vi "Config.vi"(8 "error in (no error)":errorcluster, 10 "Setting":variant, 11 "KE27XX DMM in":refnum<class "Keithley 27XX DMM.lvclass">) -> (0 "error out":errorcluster, 3 "KE27XX DMM out":refnum<class "Keithley 27XX DMM.lvclass">)   [LabVIEW 2025, in "DMM.lvlib" / "Keithley 27XX DMM.lvclass"]
uses:
  Keithley 27XX DMM.lvclass
  C:/Users/Public/Documents/Sandia National Labs/TSS Plugin/CEF.lvlibp/Node/CEF_Node.lvclass
  C:/Working copy/tss/Plugin/Engines/DMM/DMM Instrument/DMM Instrument.lvclass
  C:/Users/Public/Documents/Sandia National Labs/TSS Plugin/Abstract Engine.lvlibp/Abstract Instrument/Abstract Instrument.lvclass
  DMM configuration/DMM configuration.lvclass
  Keithley 27XX DMM.lvclass/Keithley 27XX DMM.ctl
  DMM configuration/DMM configuration.lvclass/DMM configuration.ctl
  DMM Channel/DMM Channel.lvclass
  Users/Public/Documents/Sandia National Labs/TSS Plugin/Abstract Engine.lvlibp/Abstract Instrument/Channel.ctl
  Users/Public/Documents/Sandia National Labs/TSS Plugin/Abstract Engine.lvlibp/Channel configuration/Channel configuration.lvclass
  DMM configuration/Read DMM Setting.vi
  Users/Public/Documents/Sandia National Labs/TSS Plugin/CEF.lvlibp/Node/ReadChildren.vi
  Users/Public/Documents/Sandia National Labs/TSS Plugin/Abstract Engine.lvlibp/Channel configuration/Read Channel Setting.vi
  Users/Public/Documents/Sandia National Labs/TSS Plugin/CEF.lvlibp/Node/CEF_Node.lvclass
  Users/Public/Documents/Sandia National Labs/TSS Plugin/CEF.lvlibp/serializable configuration/CEF_serializable configuration.lvclass
  <instrlib>/Keithley 27XX/Keithley 27XX.lvlib
  Users/Public/Documents/Sandia National Labs/TSS Plugin/Abstract Engine.lvlibp/Abstract Instrument/Abstract Instrument.lvclass
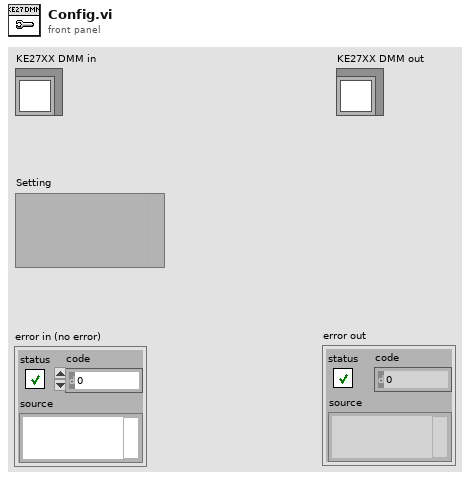
[diagram p1: front panel]
types:
  T1 = typedef "DMM.lvlib/DMM configuration.lvclass/DMM Setting.ctl" = cluster{"Function":string, "CurrentSource":string, "Resolution":string, "Range":dbl}
  T2 = typedef "Abstract Engine.lvlibp/Abstract Instrument.lvclass/Channel.ctl" = cluster{"Alias":string, "DataType":enum16{"Anaolg Input", "Waveform"}, "Unit":enum16{"---", "V", "A", "Ohm", "Hz", "uF", "degC", "deg"}, "Upper limit":dbl, "Lower limit":dbl, "Measurement":variant}
  T3 = typedef "Abstract Engine.lvlibp/Channel configuration.lvclass/Default Channel.ctl" = cluster{"Address":string, "SW Alias":string, "Enabled":bool, "Type":string, "Description":string}
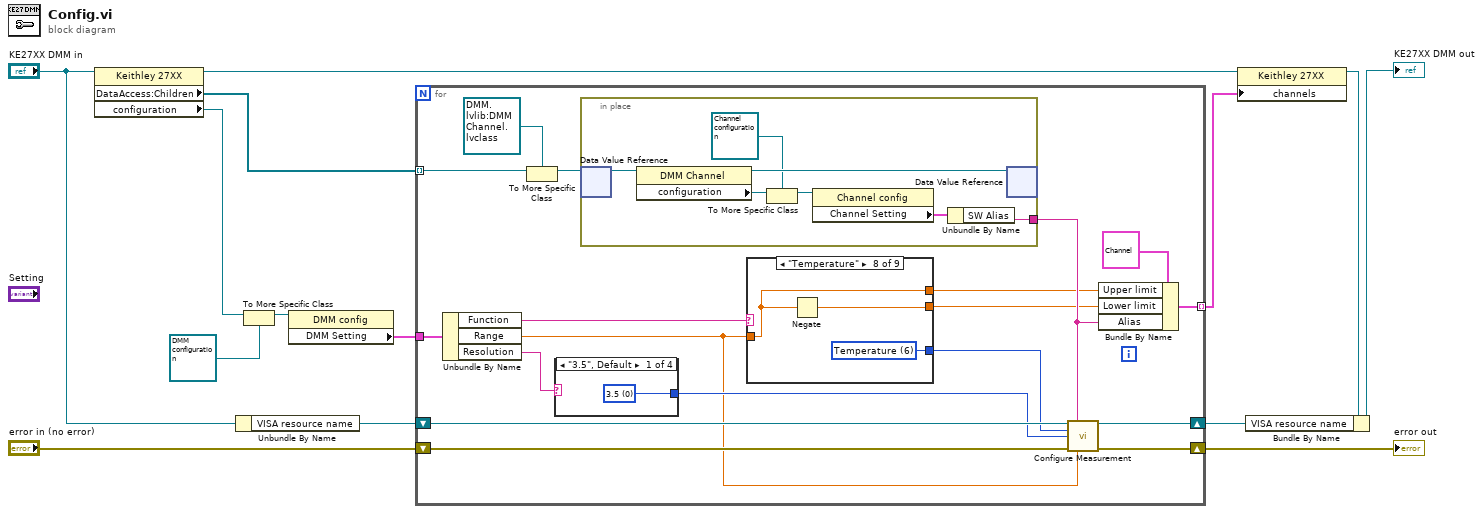
[diagram p0: block diagram]
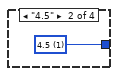
[diagram p2: hidden frame]
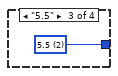
[diagram p3: hidden frame]
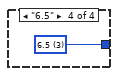
[diagram p4: hidden frame]
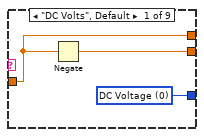
[diagram p5: hidden frame]
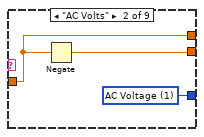
[diagram p6: hidden frame]
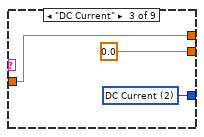
[diagram p7: hidden frame]
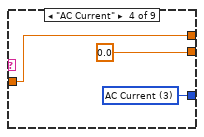
[diagram p8: hidden frame]
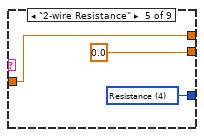
[diagram p9: hidden frame]
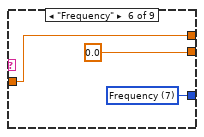
[diagram p10: hidden frame]
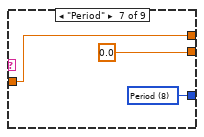
[diagram p11: hidden frame]
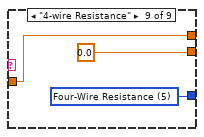
[diagram p12: hidden frame]
diagram:
  n1 = property class="Keithley 27XX"(reference="KE27XX DMM in") -> (reference out=w9:refnum<class "Keithley 27XX DMM.lvclass">, "DataAccess:Children"=w7:refnum<data-value>[], "configuration"=w8:refnum<class "CEF_serializable configuration.lvclass">)  [unwired: 1 in, 1 out]
  n2 = Unbundle By Name("KE27XX DMM in") -> ("VISA resource name"=w14:refnum<visa-resource-name>)
  n3 = To More Specific Class(target class=refnum<class "DMM configuration.lvclass"> refnum ("DMM.lvlib:DMM configuration.lvclass"), reference=w8) -> (specific class reference=w10:refnum<class "DMM configuration.lvclass">)  [unwired: 1 in, 1 out]
  n4 = property class="DMM config"(reference=w10) -> ("DMM Setting"=w5:T1)  [unwired: 1 in, 2 out]
  n5 = for {
    tunnel: w5 -> [w26]
    shift-right: [w28] -> w11
    shift-left: w14 -> [w32]
    shift-right: [w29] -> w13
    shift-left: "error in (no error)" -> [w27]
    tunnel: w7 -> [w25] mode=indexing
    tunnel: [w20] -> w1 mode=indexing
    n6 = Unbundle By Name(w26) -> ("Function"=w23:string, "Range"=w18:dbl, "Resolution"=w19:string)
    n7 = To More Specific Class(target class=refnum<data-value> refnum ("data value reference"), reference=w25) -> (specific class reference=w24:refnum<data-value>)  [unwired: 1 in, 1 out]
    n8 = case shown="\"3.5\", Default" w19 {
      tunnel: [w40 w41 w42 w43] -> w30
      frame "3.5", Default {
        w40 = u16 0 items=["3.5", "4.5", "5.5", "6.5"] ("Resolution (3: 6.5 Digits)")
      }
      frame "4.5" {
        w41 = u16 1 items=["3.5", "4.5", "5.5", "6.5"] ("Resolution (3: 6.5 Digits)")
      }
      frame "5.5" {
        w42 = u16 2 items=["3.5", "4.5", "5.5", "6.5"] ("Resolution (3: 6.5 Digits)")
      }
      frame "6.5" {
        w43 = u16 3 items=["3.5", "4.5", "5.5", "6.5"] ("Resolution (3: 6.5 Digits)")
      }
    }
    n9 = in-place {
      in-place-border: [w35] -> w21
      n10 = in-place-dvr #1(w24) -> (w39:refnum<class "DMM Channel.lvclass">)  [unwired: 1 out]
      n11 = property class="DMM Channel"(reference=w39) -> (reference out=w38:refnum<class "DMM Channel.lvclass">, "configuration"=w37:refnum<class "CEF_serializable configuration.lvclass">)  [unwired: 1 in, 1 out]
      n12 = To More Specific Class(target class=refnum<class "Channel configuration.lvclass"> refnum ("Abstract Engine.lvlibp:Channel config"), reference=w37) -> (specific class reference=w36:refnum<class "Channel configuration.lvclass">)  [unwired: 1 in, 1 out]
      n13 = property class="Channel config"(reference=w36) -> ("Channel Setting"=w34:T3)  [unwired: 1 in, 2 out]
      n14 = Unbundle By Name(w34) -> ("SW Alias"=w35:string)
      n15 = in-place-dvr #1(w38) -> ()  [unwired: 2 out]
    }
    n16 = case shown="\"Temperature\"" w23 {
      tunnel: [w46 w49 w52 w55 w58 w61 w64 w67 w70] -> w31
      tunnel: w18 -> [w45 w48 w51 w54 w57 w60 w63 w66 w69]
      tunnel: [w45 w48 w51 w54 w57 w60 w63 w66 w69] -> w17
      tunnel: [w44 w47 0.0 0.0 0.0 0.0 0.0 w65 0.0] -> w16
      frame "DC Volts", Default {
        w46 = u16 0 items=["DC Voltage", "AC Voltage", "DC Current", "AC Current", "Resistance", "Four-Wire Resistance", "Temperature", "Frequency", "Period", "Continuity"] ("Function (0: DC Voltage)")
        n17 = Negate(x=w45) -> (-x=w44:dbl)
      }
      frame "AC Volts" {
        w49 = u16 1 items=["DC Voltage", "AC Voltage", "DC Current", "AC Current", "Resistance", "Four-Wire Resistance", "Temperature", "Frequency", "Period", "Continuity"] ("Function (0: DC Voltage)")
        n18 = Negate(x=w48) -> (-x=w47:dbl)
      }
      frame "DC Current" {
        w52 = u16 2 items=["DC Voltage", "AC Voltage", "DC Current", "AC Current", "Resistance", "Four-Wire Resistance", "Temperature", "Frequency", "Period", "Continuity"] ("Function (0: DC Voltage)")
      }
      frame "AC Current" {
        w55 = u16 3 items=["DC Voltage", "AC Voltage", "DC Current", "AC Current", "Resistance", "Four-Wire Resistance", "Temperature", "Frequency", "Period", "Continuity"] ("Function (0: DC Voltage)")
      }
      frame "2-wire Resistance" {
        w58 = u16 4 items=["DC Voltage", "AC Voltage", "DC Current", "AC Current", "Resistance", "Four-Wire Resistance", "Temperature", "Frequency", "Period", "Continuity"] ("Function (0: DC Voltage)")
      }
      frame "Frequency" {
        w61 = u16 7 items=["DC Voltage", "AC Voltage", "DC Current", "AC Current", "Resistance", "Four-Wire Resistance", "Temperature", "Frequency", "Period", "Continuity"] ("Function (0: DC Voltage)")
      }
      frame "Period" {
        w64 = u16 8 items=["DC Voltage", "AC Voltage", "DC Current", "AC Current", "Resistance", "Four-Wire Resistance", "Temperature", "Frequency", "Period", "Continuity"] ("Function (0: DC Voltage)")
      }
      frame "Temperature" {
        w67 = u16 6 items=["DC Voltage", "AC Voltage", "DC Current", "AC Current", "Resistance", "Four-Wire Resistance", "Temperature", "Frequency", "Period", "Continuity"] ("Function (0: DC Voltage)")
        n19 = Negate(x=w66) -> (-x=w65:dbl)
      }
      frame "4-wire Resistance" {
        w70 = u16 5 items=["DC Voltage", "AC Voltage", "DC Current", "AC Current", "Resistance", "Four-Wire Resistance", "Temperature", "Frequency", "Period", "Continuity"] ("Function (0: DC Voltage)")
      }
    }
    n20 = call <instrlib>:"Configure Measurement.vi"("VISA resource name"=w32, "Scan List (Empty)"=w21, "Function (0: DC Voltage)"=w31, "Resolution (3: 6.5 Digits)"=w30, "error in (no error)"=w27, "Manual Range (10)"=w18) -> ("VISA resource name out"=w28:refnum<visa-resource-name>, "error out"=w29:errorcluster)  [unwired: 8 in]
    n21 = Bundle By Name(cluster=T2 {"Alias"="ch0", "DataType"=enum."Anaolg Input", "Unit"=enum."V", "Upper limit"=10.0, "Lower limit"=-10.0, "Measurement"=variant} ("Channel"), "Upper limit"=w17, "Lower limit"=w16, "Alias"=w21) -> (w20:T2)
  }
  "error out" <- w13
  n22 = property class="Keithley 27XX"(reference=w9, "channels"=w1) -> (reference out=w3:refnum<class "Keithley 27XX DMM.lvclass">)  [unwired: 1 in, 1 out]
  n23 = Bundle By Name(cluster=w3, "VISA resource name"=w11) -> (→"KE27XX DMM out":refnum<class "Keithley 27XX DMM.lvclass">)
